vi "Launch Cylinder Actor.vi"(5 "DedicatedEnQrs":refnum<queue>, 6 "SHVs":T1, 7 "Name":string, 8 "error in (no error)":errorcluster, 9 "Interlock Chain":refnum<class "Interlock Chain.lvclass">, 10 "Caller Actor in":refnum<class "Actor.lvclass">, 11 "Cylinder in":refnum<class "Cylinder.lvclass">) -> (0 "error out":errorcluster, 3 "Caller-To-Actor Enqueuer":refnum<class "Message Enqueuer.lvclass">)   [LabVIEW 2015, in "cRIO-Carbondioxide.lvlib" / "CO2-Actor.lvlib" / "Cylinder.lvclass"]
uses:
  Cylinder.lvclass
  <vilib>/ActorFramework/Message Enqueuer/Message Enqueuer.lvclass
  <vilib>/ActorFramework/Actor/Actor.lvclass
  Interlocks/Interlock Chain/Interlock Chain.lvclass
  Controls/Dedicated Enqueuers.ctl
  Cylinder.lvclass/Cylinder.ctl
  CO2 Actor/CO2 Actor.lvclass
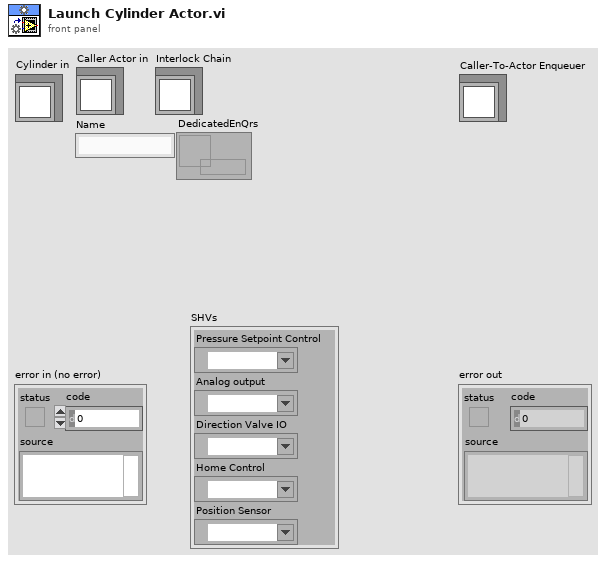
[diagram p1: front panel]
types:
  T1 = cluster{"Pressure Setpoint Control ":refnum<k21>, "Analog output":refnum<k21>, "Direction Valve IO":refnum<k21>, "Home Control":refnum<k21>, "Position Sensor":refnum<k21>}
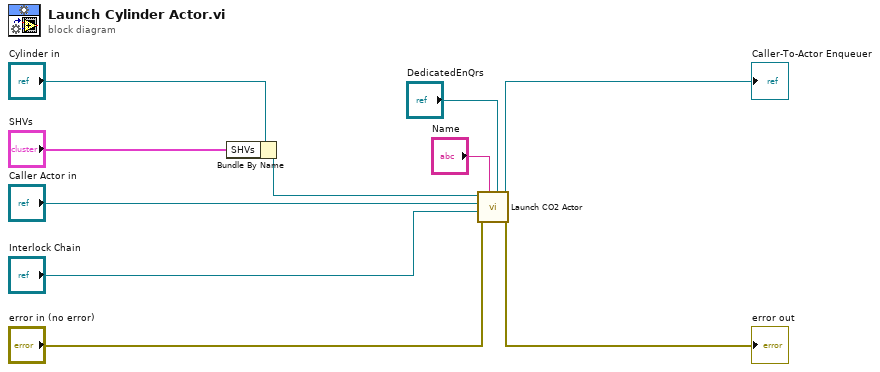
[diagram p0: block diagram]
diagram:
  n1 = Bundle By Name(cluster="Cylinder in", "SHVs"="SHVs") -> (w4:refnum<class "Cylinder.lvclass">)
  n2 = call "Launch CO2 Actor.vi"("DedicatedEnQrs"="DedicatedEnQrs", "Name"="Name", "error in (no error)"="error in (no error)", "Interlock Chain"="Interlock Chain", "Caller Actor in"="Caller Actor in", "CO2 Actor in"=w4) -> ("error out"=→"error out":errorcluster, "Caller-To-Actor Enqueuer"=→"Caller-To-Actor Enqueuer":refnum<class "Message Enqueuer.lvclass">)  [unwired: 4 in]
